vi "Helper - HDI Start Position.vi"() -> ()   [LabVIEW 2011]
uses:
  Orient3d Class/Type Definitions/Quaternion.ctl
  Gantry Class/Gantry Class.lvclass
  Vec3d Class/Vec3d Class.lvclass
  Orient3d Class/Orient3d Class.lvclass
panel:
  in  "Tab Control":enum32{"Control", "Results"}(tab)
  out "error out":errorcluster
  out "preview":T1(plugin-control)
  out "Current Position":cluster{"X":dbl, "Y":dbl, "Z":dbl}
  in  "Slot Number":u32
  in  "Capture":bool
  in  "Config Folder":path=path "C:/Users/Husker/Desktop/gantry/Config"
  out "Orientation":T2
  out "Center":cluster{"X":dbl, "Y":dbl, "Z":dbl}
  out "Residual":dbl
  out "Measured Positions":cluster{"X":dbl, "Y":dbl, "Z":dbl}[](array[cluster])
  out "Known Positions":cluster{"X":dbl, "Y":dbl, "Z":dbl}[](array[cluster])
  out "DoCapture":bool
  # "Set this to the appropriate slot number before running"
  # "Press this button after \ncentering the fiducial in the image"
  # "After aquiring positions, place these results in\npart_location.ini under the HDI heading"
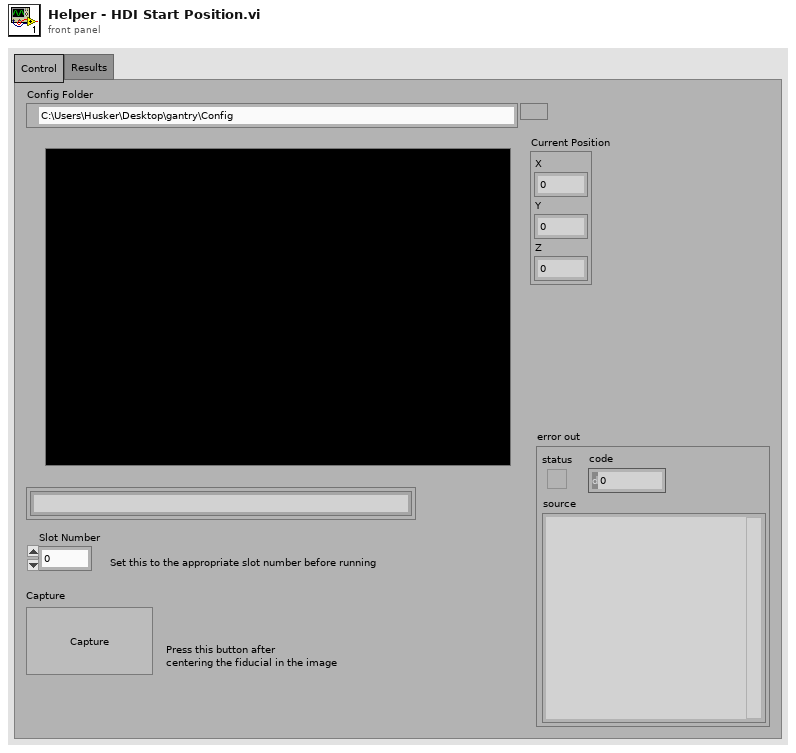
[diagram p1: front panel]
types:
  T1 = typedef "IMAQ Image.ctl" = refnum<image>
  T2 = typedef "Quaternion.ctl" = cluster{"x":dbl, "y":dbl, "z":dbl, "w":dbl}
  T3 = typedef "Image Type" = u32
  T4 = typedef "Position_Orientation.ctl" = cluster{"Center":refnum<class "Vec3d Class.lvclass">, "Orientation":refnum<class "Orient3d Class.lvclass">}
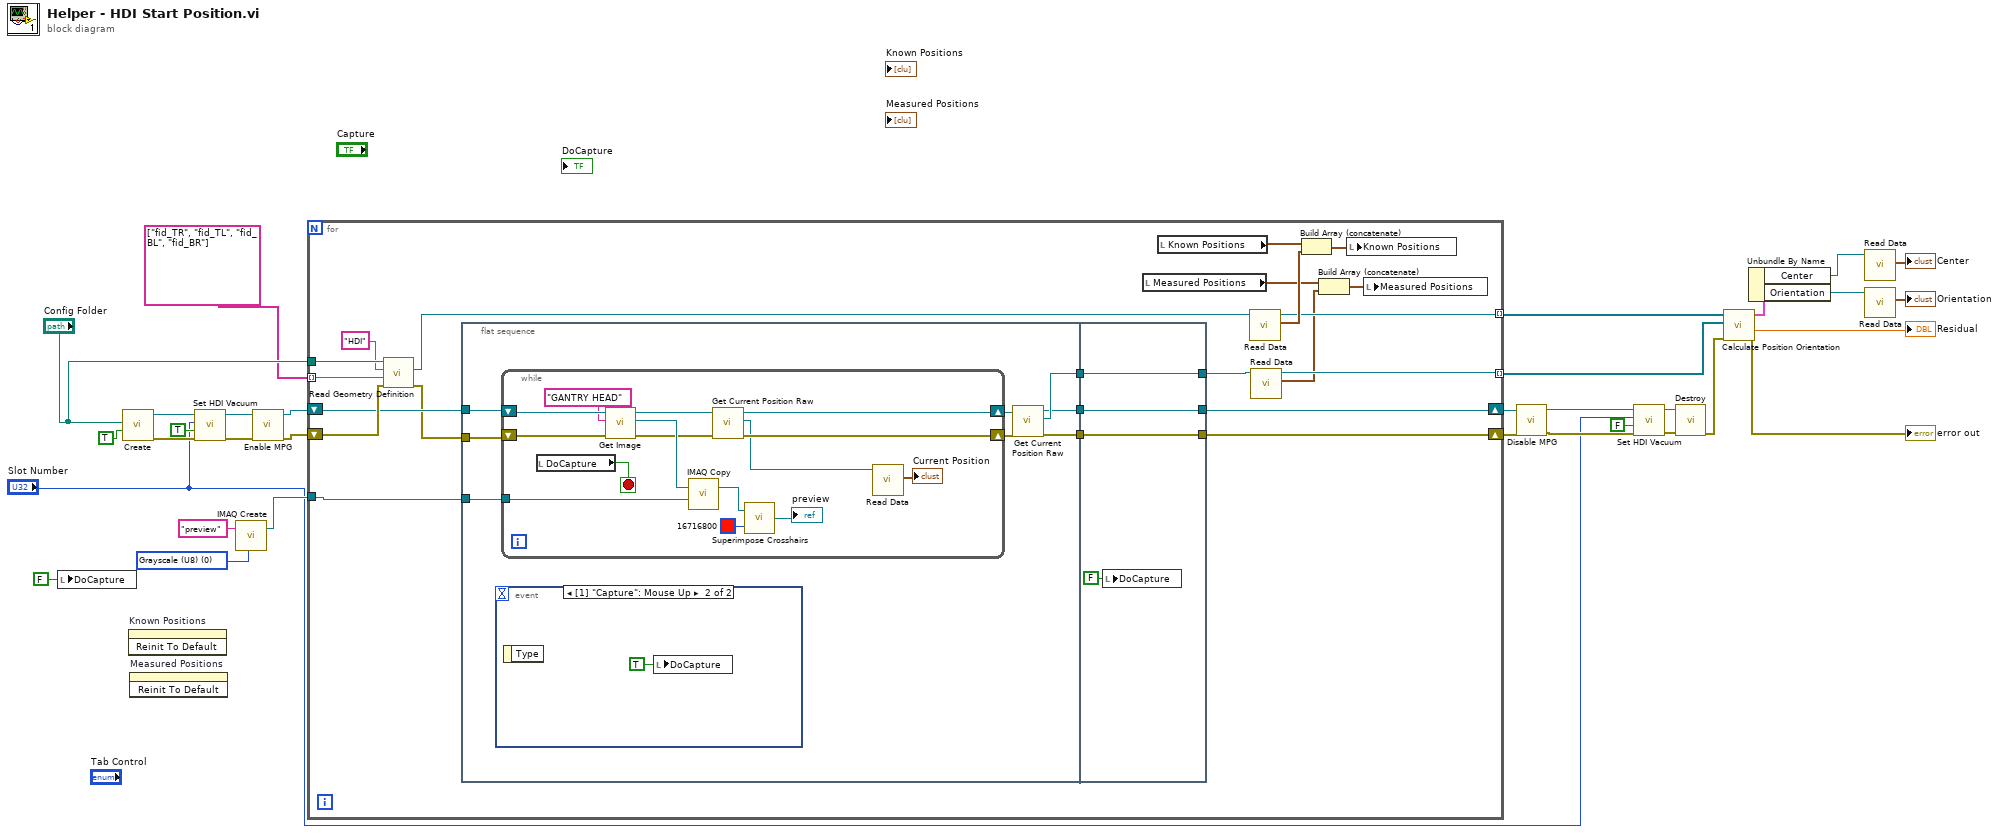
[diagram p0: block diagram]
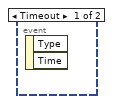
[diagram p2: hidden frame]
diagram:
  w19 = T3 0 items=["Grayscale (U8)", "Grayscale (I16)", "Grayscale (SGL)", "Complex (CSG)", "RGB (U32)", "HSL (U32)", "RGB (U64)", "Grayscale (U16)"] ("Image Type")
  n1 = local write "DoCapture"(FALSE ("DoCapture")) -> ()
  n2 = call "Create.vi"("HOME?"=TRUE, "Config Folder"="Config Folder") -> ("error out"=w27:errorcluster, "Gantry out"=w28:refnum<class "Gantry Class.lvclass">)  [unwired: 8 in]
  n3 = invoke on="Known Positions" class="Arr (strict)" method="Reinit To Default"() -> ()  [unwired: 3 in, 3 out]
  n4 = invoke on="Measured Positions" class="Arr (strict)" method="Reinit To Default"() -> ()  [unwired: 3 in, 3 out]
  n5 = call-dynamic "Set HDI Vacuum.vi"("error in"=w27, "On/Off"=TRUE, "Slot Number"="Slot Number", "Gantry in"=w28) -> ("error out"=w23:errorcluster, "Gantry out"=w25:refnum<class "Gantry Class.lvclass">)  [unwired: 6 in]
  n6 = call "IMAQ Create"("Image Name"="preview", "Image Type"=w19) -> ("New Image"=w17:T1)  [unwired: 3 in, 1 out]
  n7 = call-dynamic "Enable MPG.vi"("error in (no error)"=w23, "Gantry Class in"=w25) -> ("error out"=w22:errorcluster, "Gantry Class out"=w24:refnum<class "Gantry Class.lvclass">)  [unwired: 8 in]
  n8 = for {
    tunnel: "Config Folder" -> [w54]
    tunnel: string[] ["fid_TR", "fid_TL", "fid_BL", "fid_BR"] -> [w52] mode=indexing
    tunnel: [w38] -> w16 mode=indexing
    tunnel: [w36] -> w15 mode=indexing
    shift-right: [w48] -> w21
    shift-left: w24 -> [w50]
    shift-right: [w47] -> w20
    shift-left: w22 -> [w51]
    tunnel: w17 -> [w43]
    n9 = call "Read Geometry Definition.vi"("error in"=w51, "Feature"=w52, "Part"="HDI", "Config Location"=w54) -> ("error out"=w49:errorcluster, "Feature Coordinates"=w42:refnum<class "Vec3d Class.lvclass">)  [unwired: 6 in]
    n10 = flat-sequence {
      tunnel: w50 -> [w62]
      tunnel: w49 -> [w61]
      tunnel: [w58] -> w46
      tunnel: [w57] -> w45
      tunnel: [w56] -> w44
      tunnel: w43 -> [w55]
      tunnel: [w80] -> w47
      tunnel: [w81] -> w48
      tunnel: [w82] -> w37
      tunnel: w46 -> [w82]
      tunnel: w45 -> [w81]
      tunnel: w44 -> [w80]
      frame #0 {
        n11 = event shown="[1] \"Capture\": Mouse Up" {
          selector: _ -> [_ _]
          dyn-events: _ -> [_ _]
          timeout: _ -> [_ _]
          event Timeout {
            n12 = event-data() -> ()  [unwired: 1 in, 2 out]
          }
          event "Capture": Mouse Up {
            n13 = event-data() -> ()  [unwired: 1 in, 1 out]
            n14 = local write "DoCapture"(TRUE ("DoCapture")) -> ()
          }
        }
        n15 = while {
          shift-right: [w69] -> w60
          shift-left: w61 -> [w76]
          shift-right: [w70] -> w59
          shift-left: w62 -> [w77]
          tunnel: w55 -> [w74]
          stop <- w78 stop-if-true
          n16 = local read "DoCapture"() -> (w78:bool)
          n17 = call-dynamic "Get Image.vi"("error in"=w76, "Camera Name"="GANTRY HEAD", "Gantry in"=w77) -> ("error out"=w71:errorcluster, "Image Out"=w73:T1, "Gantry out"=w72:refnum<class "Gantry Class.lvclass">)  [unwired: 6 in]
          n18 = call "IMAQ Copy"("Image Dst"=w74, "Image Src"=w73) -> ("Image Dst Out"=w65:T1)  [unwired: 4 in, 1 out]
          n19 = call-dynamic "Get Current Position Raw.vi"("error in (no error)"=w71, "Gantry Class in"=w72) -> ("error out"=w69:errorcluster, "Vec3d Class out"=w68:refnum<class "Vec3d Class.lvclass">, "Gantry Class out"=w70:refnum<class "Gantry Class.lvclass">)  [unwired: 7 in]
          n20 = call "Superimpose Crosshairs.vi"("Grid Line Color"=u32 16716800, "Refnum in"=w65) -> ("Refnum out"=→"preview":T1)
          n21 = call-dynamic "Read Data.vi"("Vec3d Class in"=w68) -> ("Data"=→"Current Position":cluster{"X":dbl, "Y":dbl, "Z":dbl})  [unwired: 8 in, 2 out]
        }
        n22 = call-dynamic "Get Current Position Raw.vi"("error in (no error)"=w60, "Gantry Class in"=w59) -> ("error out"=w56:errorcluster, "Vec3d Class out"=w58:refnum<class "Vec3d Class.lvclass">, "Gantry Class out"=w57:refnum<class "Gantry Class.lvclass">)  [unwired: 7 in]
      }
      frame #1 {
        n23 = local write "DoCapture"(FALSE ("DoCapture")) -> ()
      }
    }
    n24 = local read "Measured Positions"() -> (w35:cluster{"X":dbl, "Y":dbl, "Z":dbl}[])
    n25 = local read "Known Positions"() -> (w41:cluster{"X":dbl, "Y":dbl, "Z":dbl}[])
    n26 = call-dynamic "Read Data.vi"("Vec3d Class in"=w42) -> ("Data"=w40:cluster{"X":dbl, "Y":dbl, "Z":dbl}, "Vec3d Class out"=w38:refnum<class "Vec3d Class.lvclass">)  [unwired: 8 in, 1 out]
    n27 = call-dynamic "Read Data.vi"("Vec3d Class in"=w37) -> ("Data"=w33:cluster{"X":dbl, "Y":dbl, "Z":dbl}, "Vec3d Class out"=w36:refnum<class "Vec3d Class.lvclass">)  [unwired: 8 in, 1 out]
    n28 = Build Array (concatenate)(w41, w40) -> (w39:cluster{"X":dbl, "Y":dbl, "Z":dbl}[])
    n29 = Build Array (concatenate)(w35, w33) -> (w34:cluster{"X":dbl, "Y":dbl, "Z":dbl}[])
    n30 = local write "Known Positions"(w39) -> ()
    n31 = local write "Measured Positions"(w34) -> ()
  }
  n32 = call-dynamic "Disable MPG.vi"("error in (no error)"=w20, "Gantry Class in"=w21) -> ("error out"=w4:errorcluster, "Gantry Class out"=w6:refnum<class "Gantry Class.lvclass">)  [unwired: 8 in]
  n33 = call-dynamic "Set HDI Vacuum.vi"("error in"=w4, "On/Off"=FALSE, "Slot Number"="Slot Number", "Gantry in"=w6) -> ("error out"=w3:errorcluster, "Gantry out"=w5:refnum<class "Gantry Class.lvclass">)  [unwired: 6 in]
  n34 = call "Destroy.vi"("error in"=w3, "Gantry Class in"=w5) -> ("error out"=w13:errorcluster)  [unwired: 9 in]
  n35 = call "Calculate Position Orientation.vi"("error in"=w13, "Measured Global Positions"=w15, "Known Local Positions"=w16) -> ("error out"=→"error out":errorcluster, "Residual"=→"Residual":dbl, "PositionOrientation"=w11:T4)  [unwired: 6 in]
  n36 = Unbundle By Name(w11) -> ("Center"=w10:refnum<class "Vec3d Class.lvclass">, "Orientation"=w8:refnum<class "Orient3d Class.lvclass">)
  n37 = call-dynamic "Read Data.vi"("Vec3d Class in"=w10) -> ("Data"=→"Center":cluster{"X":dbl, "Y":dbl, "Z":dbl})  [unwired: 8 in, 2 out]
  n38 = call "Read Data.vi"("Orient3d in"=w8) -> ("Quaternion"=→"Orientation":T2)  [unwired: 8 in, 2 out]
